vi "UI Initialize.vi"(8 "error in (no error)":errorcluster, 11 "UI ActorTop in":refnum<class "UIActorTop.lvclass">) -> (0 "error out":errorcluster, 3 "UI ActorTop out":refnum<class "UIActorTop.lvclass">)   [LabVIEW 2021, in "AbstractActorTemplate.lvlib" / "UIActorTop.lvclass"]
doc: "UI: Initialize\n2015-03-18 16:27:22\n蒋松\njiangsong@outlook.com"
uses:
  <userlib>/John_Lib/AbstractActorTemplate/AbstractActorTemplate/UIActorTop.lvclass
  <userlib>/John_Lib/AbstractActorTemplate/AbstractActorTemplate/UIActorTop.lvclass/UIActorTop.ctl
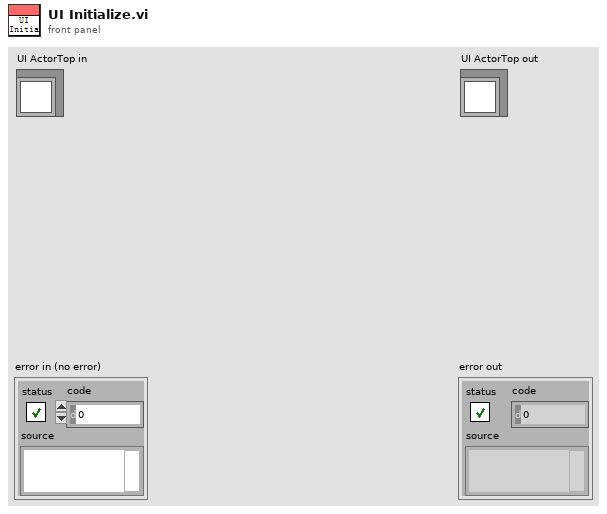
[diagram p1: front panel]
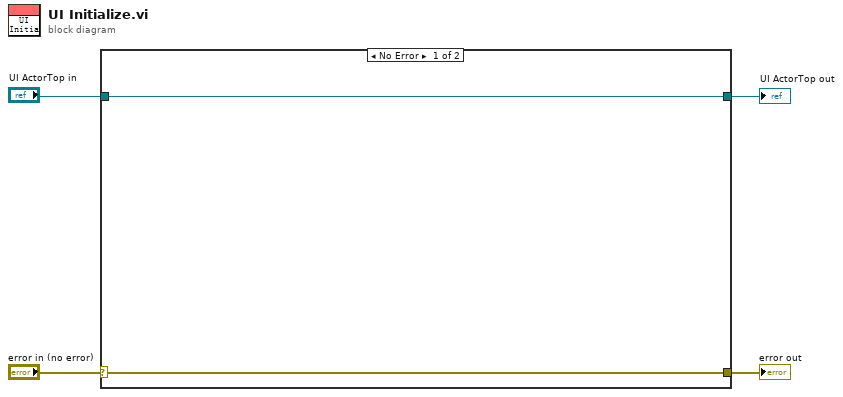
[diagram p0: block diagram]
diagram:
  n1 = case shown="No Error" "error in (no error)" {
    selector: "error in (no error)" -> [w6 w8]
    tunnel: [w6 w8] -> w3
    tunnel: [w5 w7] -> w2
    tunnel: "UI ActorTop in" -> [w5 w7]
    frame No Error {
    }
    frame Error {
    }
  }
  "error out" <- w3
  "UI ActorTop out" <- w2
